vi "Aluminum Material Properties.vi"(6 "m-nm Al":dbl, 9 "Aluminum Thickness":dbl, 10 "Energy (Heat; I^2R)":dbl, 11 "NS Base Area":dbl) -> (1 "Mass  Al":dbl, 2 "Delta Temp Change Al":dbl, 3 "Al Specfic Heat Capacity":dbl, 4 "Volume Al":dbl, 5 "Al Density":dbl, 7 "Al Thickness":dbl)   [LabVIEW 2020]
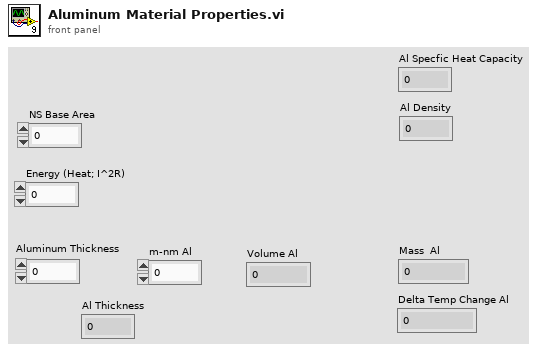
[diagram p1: front panel]
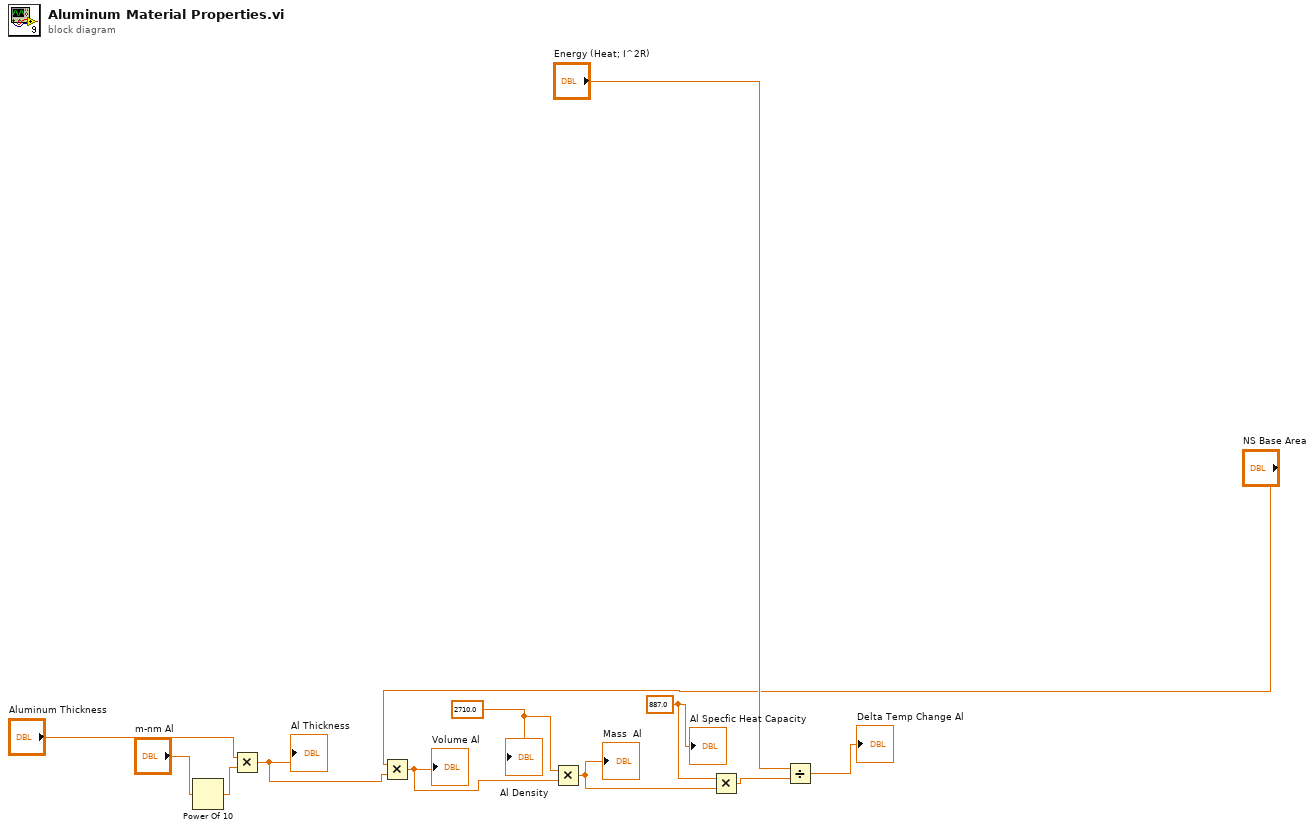
[diagram p0: block diagram]
diagram:
  w12 = 887.0 ("Silicon Specfic Heat Capacity 5")
  w5 = 2710.0 ("Silicon Density 5")
  n1 = Power Of 10(x="m-nm Al") -> (10^x=w1:dbl)
  n2 = Multiply(x="Aluminum Thickness", y=w1) -> (x*y=w4:dbl)
  "Al Thickness" <- w4
  n3 = Multiply(x="NS Base Area", y=w4) -> (x*y=w6:dbl)
  "Volume Al" <- w6
  n4 = Multiply(x=w5, y=w6) -> (x*y=w11:dbl)
  "Mass  Al" <- w11
  n5 = Multiply(x=w12, y=w11) -> (x*y=w10:dbl)
  n6 = Divide(x="Energy (Heat; I^2R)", y=w10) -> (x/y=→"Delta Temp Change Al":dbl)
  "Al Density" <- w5
  "Al Specfic Heat Capacity" <- w12
